vi "Data-Server-Handler.vi"(1 "Remote Port":u16, 2 "connection ID":refnum<k5>) -> ()   [LabVIEW 2017]
panel:
  out "Remote Port":u16
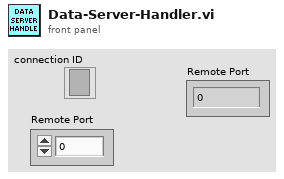
[diagram p1: front panel]
types:
  T1 = enum16{"big-endian, network order", "native, host order", "little-endian"}
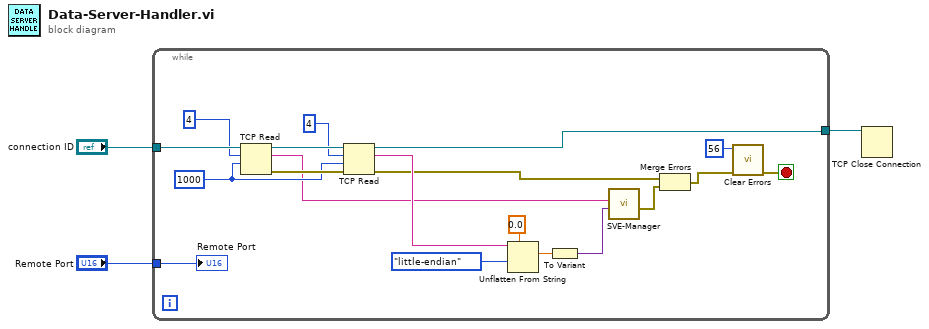
[diagram p0: block diagram]
diagram:
  n1 = while {
    tunnel: "connection ID" -> [w22]
    tunnel: "Remote Port" -> [w10]
    tunnel: [w15] -> w1
    stop <- w20 stop-if-true
    w16 = 1000 ("timeout ms (25000)")
    n2 = TCP Read(connection ID=w22, bytes to read=4, 9:w16) -> (connection ID out=w17:refnum<k5>, data out=w9:string, error out=w18:errorcluster)  [unwired: 2 in]
    n3 = TCP Read(connection ID=w17, bytes to read=4, error in (no error)=w18, 9:w16) -> (connection ID out=w15:refnum<k5>, data out=w12:string, error out=w4:errorcluster)  [unwired: 1 in]
    n4 = Unflatten From String(type=sgl 0.0 ("input 1"), binary string=w12, byte order (0:big-endian, network order)=T1."little-endian") -> (value=w8:sgl)  [unwired: 2 in, 2 out]
    n5 = To Variant(anything=w8) -> (Variant=w7:variant)
    n6 = call "SVE-Manager.vi"("Data"=w7, "DataTag"=w9) -> ("error out"=w5:errorcluster)  [unwired: 9 in]
    n7 = Merge Errors(w4, w5) -> (w6:errorcluster)
    n8 = call <vilib>:"Clear Errors.vi"("error in (no error)"=w6, "specific error code to clear (0: all)"=56) -> ("error out"=w20:errorcluster)  [unwired: 4 in, 1 out]
    "Remote Port" <- w10
  }
  n9 = TCP Close Connection(connection ID=w1) -> ()  [unwired: 2 in, 2 out]
